vi "tm_getparameter.vi"(6 "Index":i32, 8 "error in (no error)":errorcluster, 10 "Parameter":u32(ring)=1 items=["BINNING"=1, "BITS PER CHANNEL"=2, "ACTIVE VIEW INDEX"=3, "CCD MODE"=4, "SENSOR MODE"=5, "READOUT MODE"=6, "EXPOSURE TIME"=7, "CONTRAST GAIN"=8, "CONTRAST OFFSET"=9, "LIGHT MODE"=10, "SENSITIVITY"=11, "WHITE BALANCE"=12, "PHOTON IMAGING MODE"=13, "HIGH DYNAMIC RANGE MODE"=14, "TRIGGER SOURCE"=15, "TRIGGER ACTIVE"=16, "TRIGGER MODE"=17, "TRIGGER POLARITY"=18, "TRIGGER GLOBAL EXPOSURE"=19, "FIRST TRIGGER BEHAVIOR"=20, "TRIGGER TIMES"=21, "OUTPUT TRIGGER POLARITY"=22, "OUTPUT TRIGGER DELAY"=23, "OUTPUT TRIGGER PERIOD"=24, "TEMPERATURE"=25, "TEMPERATURE TARGET"=26, "SENSOR COOLER FAN"=27, "MECHANICAL SHUTTER"=28, "BACK FOCUS POSITION"=29, "FRAMEBUNDLE MODE"=30, "FRAMEBUNDLE NUMBER"=31, "LINEBUNDLE HEIGHT"=32, "TRIGGER CONNECTOR"=33, "IMAGE PIXEL TYPE"=34, "OUTPUT TRIGGER KIND"=35, "READOUT DIRECTION"=36, "CHANNEL SYNC"=37], 11 "Handle in":u32) -> (0 "error out":errorcluster, 2 "Value out":dbl, 3 "Handle out":u32)   [LabVIEW 2011]
uses:
  tmcamcon.dll
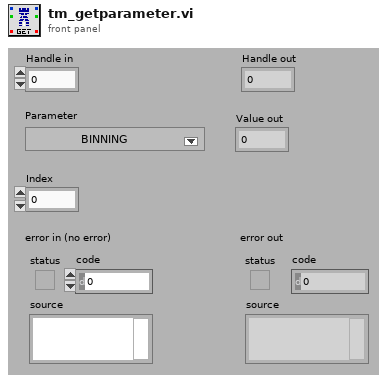
[diagram p1: front panel]
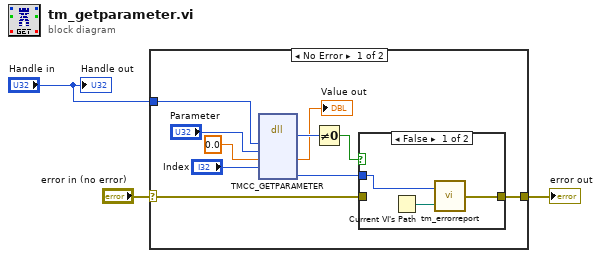
[diagram p0: block diagram]
diagram:
  n1 = case shown="No Error" "error in (no error)" {
    selector: "error in (no error)" -> [w7 w18]
    tunnel: [w4 w18] -> w2
    tunnel: "Handle in" -> [w12 _]
    frame No Error {
      n2 = dll-call lib="tmcamcon.dll" fn="TMCC_GETPARAMETER"("handle"=w12, "parameter"="Parameter", "value"=0.0, "view"="Index") -> ("return type"=w13:u32, "value"=→"Value out":dbl, "Erval"=w6:i32)  [unwired: 7 in, 2 out]
      n3 = Not Equal To 0?(x=w13) -> (x != 0?=w5:bool)
      n4 = case shown="False" w5 {
        tunnel: w7 -> [_ w17]
        tunnel: [w15 w17] -> w4
        tunnel: w6 -> [w14 _]
        frame False {
          n5 = Current VI's Path() -> (path=w16:path)
          n6 = call <userlib>:"tm_errorreport.vi"("Source"=w16, "Error"=w14) -> ("error out"=w15:errorcluster)
        }
        frame True {
        }
      }
    }
    frame Error {
    }
  }
  "error out" <- w2
  "Handle out" <- "Handle in"
